vi "Read Multiple.vi"(8 "error in (no error)":errorcluster, 10 "Symbol Names":string[](array[string]), 11 "TwinCAT ADS in":refnum<class "TwinCAT ADS.lvclass">) -> (0 "error out":errorcluster, 1 "Values":variant[](array[variant]), 3 "TwinCAT ADS out":refnum<class "TwinCAT ADS.lvclass">)   [LabVIEW 2018, in "TwinCAT ADS.lvclass"]
uses:
  TwinCAT ADS.lvclass
  TwinCAT ADS.lvclass/TwinCAT ADS.ctl
  TwinCAT.Ads
  Get From Symbol Map.vi
  Get From Symbol Map Daemon.vi
  Get Symbol Map.vi
  Format String.vi
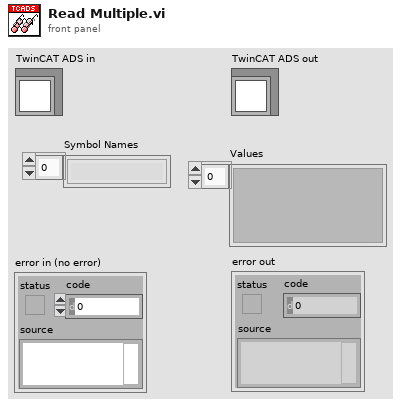
[diagram p1: front panel]
types:
  T1 = enum16{"big-endian, network order", "native, host order", "little-endian"}
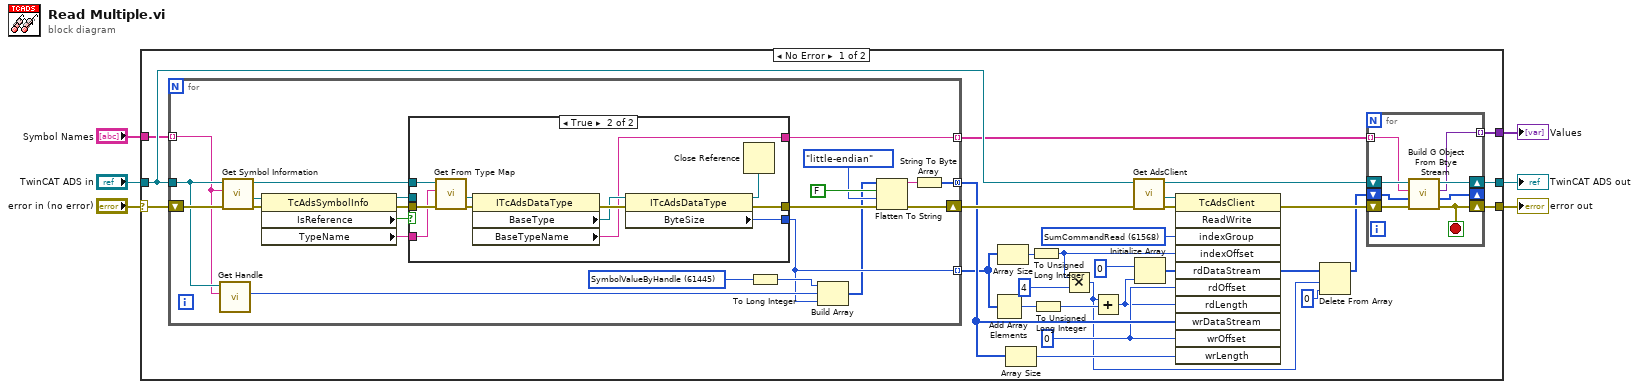
[diagram p0: block diagram]
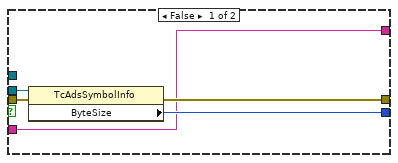
[diagram p2: hidden frame]
diagram:
  n1 = case shown="No Error" "error in (no error)" {
    selector: "error in (no error)" -> [w7 w83]
    tunnel: "Symbol Names" -> [w33 _]
    tunnel: [w32 _] -> w5
    tunnel: [w31 w83] -> w4
    tunnel: [w30 w82] -> w3
    tunnel: "TwinCAT ADS in" -> [w34 w82]
    frame No Error {
      w22 = u32 61568 items=["PlcRWIB"=16384, "PlcRWOB"=16400, "PlcRWMB"=16416, "PlcRWRB"=16432, "PlcRWDB"=16448, "SymbolTable"=61440, "SymbolName"=61441, "SymbolValue"=61442, "SymbolHandleByName"=61443, "SymbolValueByName"=61444, "SymbolValueByHandle"=61445, "SymbolReleaseHandle"=61446, "SymbolInfoByName"=61447, "SymbolVersion"=61448, "SymbolInfoByNameEx"=61449, "SymbolDownload"=61450, "SymbolUpload"=61451, "SymbolUploadInfo"=61452, "SymbolNote"=61456, "IOImageRWIB"=61472, "IOImageRWIX"=61473, "IOImageRWOB"=61488, "IOImageRWOX"=61489, "IOImageClearI"=61504, "IOImageClearO"=61520, "SumCommandRead"=61568, "SumCommandWrite"=61569, "SumCommandReadWrite"=61570, "SumCommandReadEx"=61571, "SumCommandReadEx2"=61572, "SumCommandAddDevNote"=61573, "SumCommandDelDevNote"=61574, "DeviceData"=61696] ("SumCommandRead")
      w25 = 0 ("wrOffset")
      n2 = for {
        tunnel: w33 -> [w62] mode=indexing
        tunnel: [w51] -> w11 mode=indexing
        tunnel: [w50] -> w27 mode=indexing
        shift-right: [w48] -> w35
        shift-left: w7 -> [w64]
        tunnel: [w47] -> w29 mode=concatenating
        tunnel: w34 -> [w63]
        w54 = u32 61445 items=["PlcRWIB"=16384, "PlcRWOB"=16400, "PlcRWMB"=16416, "PlcRWRB"=16432, "PlcRWDB"=16448, "SymbolTable"=61440, "SymbolName"=61441, "SymbolValue"=61442, "SymbolHandleByName"=61443, "SymbolValueByName"=61444, "SymbolValueByHandle"=61445, "SymbolReleaseHandle"=61446, "SymbolInfoByName"=61447, "SymbolVersion"=61448, "SymbolInfoByNameEx"=61449, "SymbolDownload"=61450, "SymbolUpload"=61451, "SymbolUploadInfo"=61452, "SymbolNote"=61456, "IOImageRWIB"=61472, "IOImageRWIX"=61473, "IOImageRWOB"=61488, "IOImageRWOX"=61489, "IOImageClearI"=61504, "IOImageClearO"=61520, "SumCommandRead"=61568, "SumCommandWrite"=61569, "SumCommandReadWrite"=61570, "SumCommandReadEx"=61571, "SumCommandReadEx2"=61572, "SumCommandAddDevNote"=61573, "SumCommandDelDevNote"=61574, "DeviceData"=61696] ("SumCommandRead")
        n3 = call "Get Handle.vi"("Symbol Name"=w62, "TwinCAT ADS in"=w63) -> ("Handle"=w52:i32)  [unwired: 7 in, 2 out]
        n4 = call "Get Symbol Information.vi"("error in (no error)"=w64, "Symbol Name"=w62, "TwinCAT ADS in"=w63) -> ("error out"=w61:errorcluster, ".NET Symbol Information"=w60:refnum<k24>, "TwinCAT ADS out"=w58:refnum<class "TwinCAT ADS.lvclass">)  [unwired: 6 in]
        n5 = property class="TcAdsSymbolInfo"(reference=w60, error in=w61) -> (reference out=w55:refnum<k24>, error out=w56:errorcluster, "IsReference"=w59:bool, "TypeName"=w57:string)
        n6 = case shown="True" w59 {
          tunnel: w56 -> [w70 w81]
          tunnel: w57 -> [w66 w78]
          tunnel: [w66 w71] -> w51
          tunnel: [w67 w75] -> w50
          tunnel: [w68 w73] -> w65
          tunnel: w55 -> [w69 _]
          tunnel: w58 -> [_ w72]
          frame False {
            n7 = property class="TcAdsSymbolInfo"(reference=w69, error in=w70) -> (error out=w68:errorcluster, "ByteSize"=w67:i32)  [unwired: 1 out]
          }
          frame True {
            n8 = call "Get From Type Map.vi"("error in (no error)"=w81, "Type Name"=w78, "TwinCAT ADS in"=w72) -> ("error out"=w80:errorcluster, ".NET AdsDataType"=w79:refnum<k24>)  [unwired: 6 in, 1 out]
            n9 = property class="ITcAdsDataType"(reference=w79, error in=w80) -> (error out=w77:errorcluster, "BaseType"=w76:refnum<k24>, "BaseTypeName"=w71:string)  [unwired: 1 out]
            n10 = property class="ITcAdsDataType"(reference=w76, error in=w77) -> (reference out=w74:refnum<k24>, error out=w73:errorcluster, "ByteSize"=w75:i32)
            n11 = Close Reference(reference=w74) -> ()  [unwired: 1 in, 1 out]
          }
        }
        n12 = To Long Integer(number=w54) -> (32bit integer=w53:i32)
        n13 = Build Array(w53, w52, w50) -> (w44:i32[])
        n14 = Flatten To String(anything=w44, prepend array or string size? (T)=FALSE, byte order (0:big-endian, network order)=T1."little-endian" ("Byte Order (little-endian)"), error in (no error)=w65) -> (data string=w49:string, error out=w48:errorcluster)  [unwired: 1 out]
        n15 = String To Byte Array(string=w49) -> (unsigned byte array=w47:u8[])
      }
      n16 = Add Array Elements(numeric array=w27) -> (sum=w19:i32)
      n17 = Array Size(array=w27) -> (size(s)=w26:i32)
      n18 = Array Size(array=w29) -> (size(s)=w28:i32)
      n19 = To Unsigned Long Integer(number=w26) -> (unsigned 32bit integer=w16:u32)
      n20 = To Unsigned Long Integer(number=w19) -> (unsigned 32bit integer=w15:u32)
      n21 = Multiply(x=w16, y=u32 4 ("length")) -> (x*y=w14:u32)
      n22 = Add(x=w14, y=w15) -> (x+y=w17:u32)
      n23 = call "Get AdsClient.vi"("error in (no error)"=w35, "TwinCAT ADS in"=w34) -> ("error out"=w21:errorcluster, ".NET TcAdsClient"=w20:refnum<k24>, "TwinCAT ADS out"=w12:refnum<class "TwinCAT ADS.lvclass">)  [unwired: 7 in]
      n24 = Initialize Array(u8 0, w17) -> (w23:u8[])
      n25 = invoke class="TcAdsClient" method="ReadWrite"(reference=w20, error in=w21, "indexGroup"=w22, "indexOffset"=w16, "rdDataStream"=w23, "rdOffset"=w25, "rdLength"=w17, "wrDataStream"=w29, "wrOffset"=w25, "wrLength"=w28) -> (error out=w13:errorcluster, "rdDataStream"=w9:u8[])  [unwired: 1 in, 9 out]
      n26 = Delete From Array(array=w9, length=w14, index=0) -> (array with subset deleted=w10:u8[])  [unwired: 1 out]
      n27 = for {
        tunnel: w11 -> [w40] mode=indexing
        shift-right: [w41] -> w30
        shift-left: w12 -> [w42]
        shift-right: [w36] -> w31
        shift-left: w13 -> [w43]
        tunnel: [w38] -> w32 mode=indexing
        shift-right: [w37] -> _
        shift-left: w10 -> [w39]
        stop <- w36 stop-if-true
        n28 = call "Build G Object From Btye Stream.vi"("error in (no error)"=w43, "Byte Stream in"=w39, "Type Name"=w40, "TwinCAT ADS in"=w42) -> ("error out"=w36:errorcluster, "Byte Stream out"=w37:u8[], "Value"=w38:variant, "TwinCAT ADS out"=w41:refnum<class "TwinCAT ADS.lvclass">)  [unwired: 4 in]
      }
    }
    frame Error {
    }
  }
  "error out" <- w4
  "TwinCAT ADS out" <- w3
  "Values" <- w5
